vi "LatestAPLPath.vi"(8 "Error In":errorcluster, 9 "APL Search String":T1(ring), 11 "Folder Path":path=path "\\\\itnas.appl.ge.com\\technology/Electronics/InProcess/Software/ci_builds/2015_VA_Washer") -> (0 "Error Out":errorcluster, 1 "Report text":string, 2 "Found ?":bool, 3 "File Path":path=path "\\\\itnas.appl.ge.com\\technology/Electronics/InProcess/Software/ci_builds/2015_VA_Washer/2015-03-06_03-42-38(Build-1952)/Binaries/2015VAWasher_Param_QA_Cycle_1_62_99_1.apl")   [LabVIEW 2016, in "Centauro.lvlib"]
doc: "This VI will search for the most recent version of software apls and return its path. You can search for various firware or xml apls.\n\nIf not found it will return an empty path, as well and boolean and report text."
uses:
  Projects/Centauro.lvlib
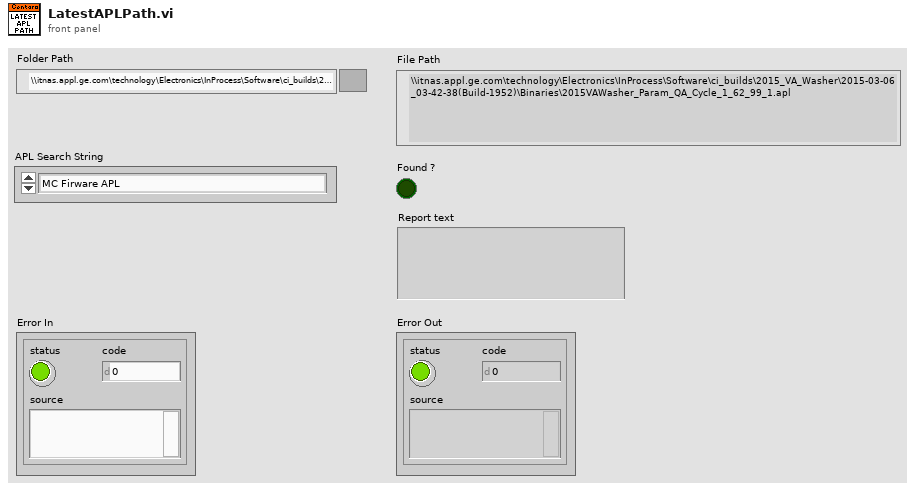
[diagram p1: front panel]
types:
  T1 = enum16{"MC Firware APL", "UI Firmware APL", "QA XML APL", "System XML", "MC ERD Definitions XML", "UI ERD Definitions XML"}
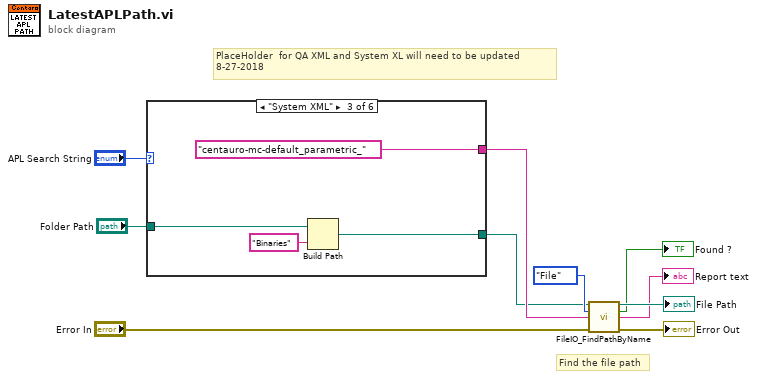
[diagram p0: block diagram]
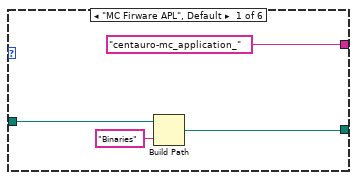
[diagram p2: hidden frame]
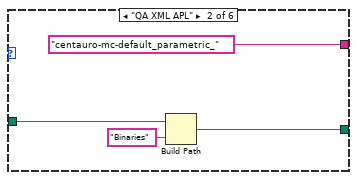
[diagram p3: hidden frame]
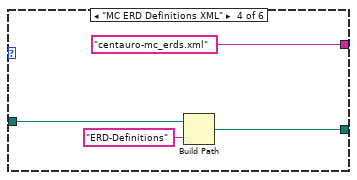
[diagram p4: hidden frame]
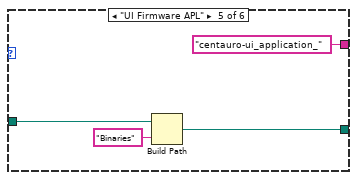
[diagram p5: hidden frame]
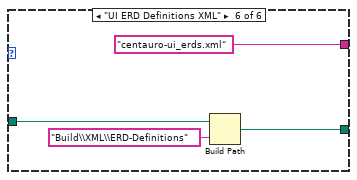
[diagram p6: hidden frame]
diagram:
  # "PlaceHolder  for QA XML and System XL will need to be updated\n8-27-2018"
  # "Find the file path"
  n1 = case shown="\"System XML\"" "APL Search String" {
    tunnel: ["centauro-mc_application_" "centauro-mc-default_parametric_" "centauro-mc-default_parametric_" "centauro-mc_erds.xml" "centauro-ui_application_" "centauro-ui_erds.xml"] -> w7
    tunnel: [w12 w16 w20 w24 w28 w31] -> w1
    tunnel: "Folder Path" -> [w13 w17 w21 w25 w29 w32]
    frame "MC Firware APL", Default {
      n2 = Build Path(base path=w13, name or relative path="Binaries") -> (appended path=w12:path)
    }
    frame "QA XML APL" {
      n3 = Build Path(base path=w17, name or relative path="Binaries") -> (appended path=w16:path)
    }
    frame "System XML" {
      n4 = Build Path(base path=w21, name or relative path="Binaries") -> (appended path=w20:path)
    }
    frame "MC ERD Definitions XML" {
      n5 = Build Path(base path=w25, name or relative path="ERD-Definitions") -> (appended path=w24:path)
    }
    frame "UI Firmware APL" {
      n6 = Build Path(base path=w29, name or relative path="Binaries") -> (appended path=w28:path)
    }
    frame "UI ERD Definitions XML" {
      n7 = Build Path(base path=w32, name or relative path="Build\\XML\\ERD-Definitions") -> (appended path=w31:path)
    }
  }
  n8 = call "FileIO_FindPathByName.vi"("Path In"=w1, "File or Folder ?"=enum16{"Folder", "File"}."File", "File/Folder Search String"=w7, "Error In"="Error In") -> ("Path Out"=→"File Path":path, "Found ?"=→"Found ?":bool, "Report Text"=→"Report text":string, "Error Out"=→"Error Out":errorcluster)  [unwired: 8 in]
